vi "BPSK QPSK Simulation.vi"() -> ()   [LabVIEW 2013]
uses:
  <vilib>/addons/Modulation/Digital/General/MT Generate Bits (Galois, PN Order).vi
  <vilib>/addons/Modulation/Digital/General/MT Generate PSK System Parameters(M).vi
  <vilib>/addons/Modulation/Digital/General/MT Generate PSK Synchronization Parameters (bit array).vi
  <vilib>/addons/Modulation/Digital/General/MT Format Eye Diagram (complex).vi
  <vilib>/addons/Modulation/niDMT.lvlib
panel:
  out "recovered bits":i32[](array[numeric])
  out "transmitted bits":i32[](array[numeric])
  in  "stop":bool
  out "eye diagram":cluster{"t0":dbl, "dt":dbl, "Y":dbl[]}[](graph)
  out "baseband waveform":cluster{"t0":dbl, "dt":dbl, "Y":dbl[]}(graph)
  out "LED Array":cluster{bool[], bool[]}
  out "constellation graph":T1(graph)
  out "measurements":T2 {"phase offset (deg)" format="%.2f"; "frequency drift (Hz)" format="%.2f"; "frequency offset (Hz)" format="%.2f"}
  out "sync found index (symbols)":dbl format="%.4f"
  in  "Eb/N0 (10 dB)":dbl(slide)=10.0 scale=0.0..500.0
  in  "modulation type":T3(ring)
  in  "pulse shaping filter (none)":T4(ring)
  in  "M-FSK (4)":i32=2 caption="M-FSK (2)"
  in  "Message Bits":i32=128 caption="Message bits"
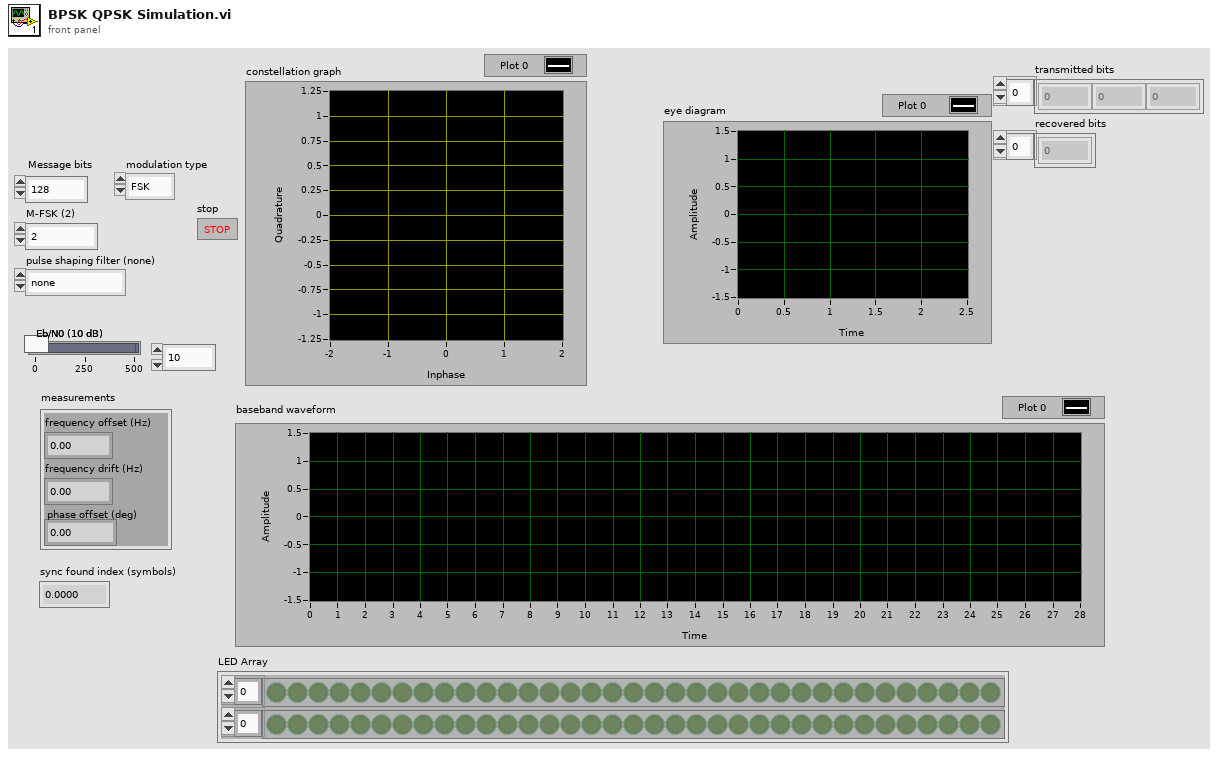
[diagram p1: front panel]
types:
  T1 = cluster{"constellation":dbl[], "oversampled data":dbl[]}[]
  T2 = cluster{"frequency offset (Hz)":dbl, "frequency drift (Hz)":dbl, "phase offset (deg)":dbl}
  T3 = enum16{"FSK", "PSK", "QAM", "MSK", "PAM", "ASK", "CPM"}
  T4 = enum16{"none", "Raised Cosine", "Root Raised Cos", "Gaussian"}
  T5 = cluster{"samples per symbol (16)":i32, "symbol map":cdb[], "differential PSK":enum16{"disable", "enable"}, "PSK type":u16}
  T6 = typedef "niAMT.lvlib/Complex Data Waveform.ctl" = cluster{"t0":dbl, "dt":dbl, "Y":cdb[]}
  T7 = cluster{"expected sync location (symbols)":i32, "sync sequence":cdb[], "sync location uncertainty (symbols)":i32, "sync indent (symbols)":i32}
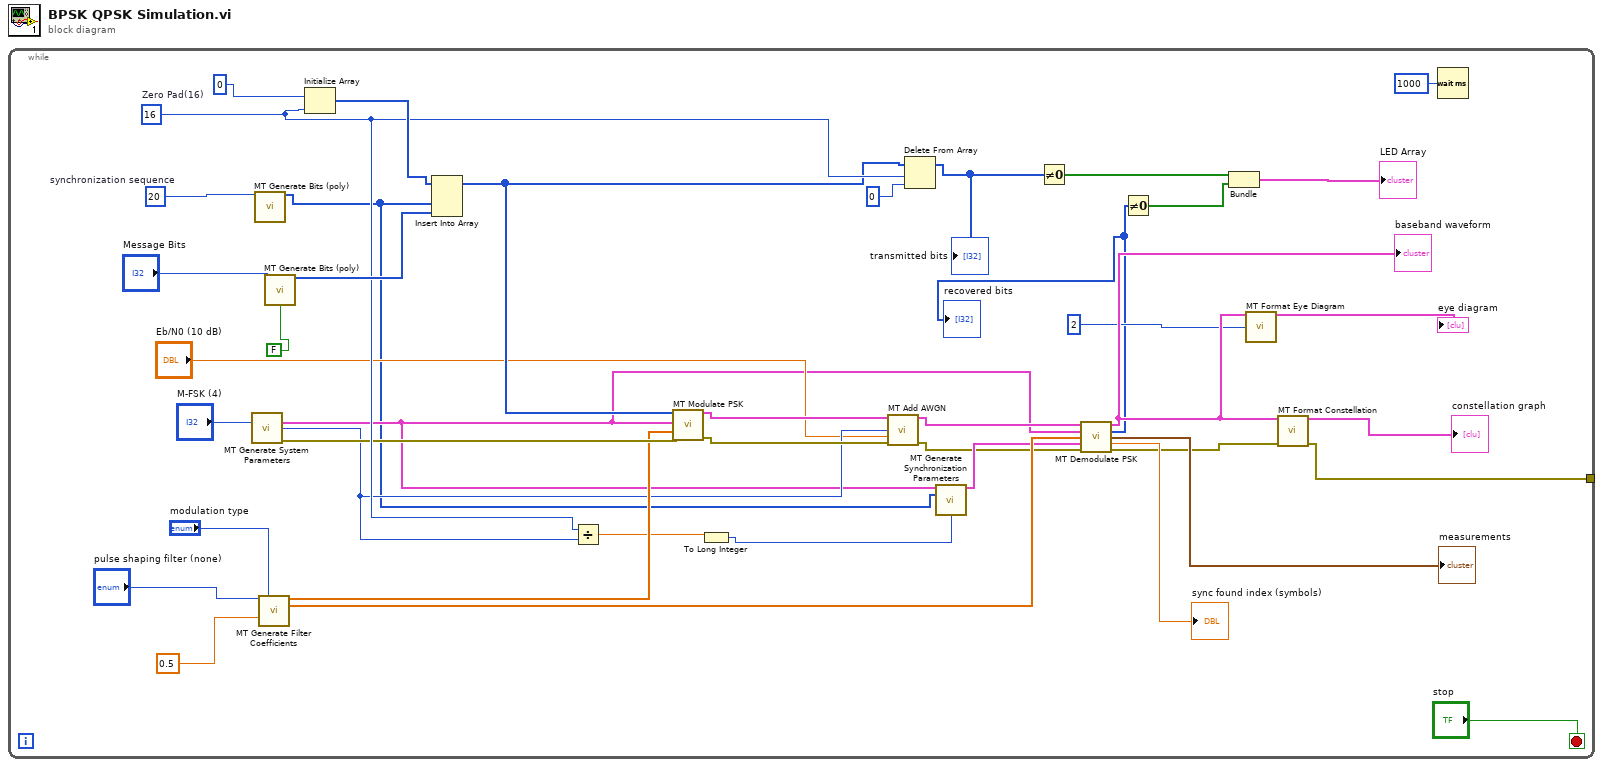
[diagram p0: block diagram]
diagram:
  n1 = while {
    tunnel: [w3] -> _
    stop <- "stop" stop-if-true
    w40 = 20  # synchronization sequence
    w28 = 16  # Zero Pad(16)
    n2 = call-poly <vilib>:"MT Generate System Parameters.vi"("M-PSK (4)"="M-FSK (4)") -> ("PSK system parameters"=w16:T5, "bits per symbol"=w22:i32, "error out"=w27:errorcluster)  [unwired: 12 in]
    n3 = call-poly <vilib>:"MT Generate Bits (poly).vi"("total bits (128)"=w40) -> ("output bit stream"=w15:i8[])  [unwired: 12 in, 2 out]
    n4 = call <vilib>:"MT Generate Filter Coefficients.vi"("pulse shaping filter (none)"="pulse shaping filter (none)", "modulation type"="modulation type", "filter parameter"=0.5) -> ("pulse shaping filter coefficients"=w26:dbl[], "matched filter coefficients"=w19:dbl[])  [unwired: 10 in, 1 out]
    n5 = call-poly <vilib>:"MT Generate Bits (poly).vi"("total bits (128)"="Message Bits", "reset? (T)"=FALSE) -> ("output bit stream"=w37:i8[])  [unwired: 11 in, 2 out]
    n6 = Initialize Array "Initialize Array"(0, w28) -> (w41:i32[])
    n7 = Insert Into Array "Insert Into Array"(array=w41, new element #1=w15, new element #2=w37) -> (w24:i32[])  [unwired: 1 in]
    n8 = Divide(x=w28, y=w22) -> (x/y=w18:dbl)
    n9 = call <vilib>:"MT Modulate PSK.vi"("input bit stream"=w24, "PSK system parameters"=w16, "pulse shaping filter coefficients"=w26, "error in (no error)"=w27) -> ("output complex waveform"=w25:T6, "error out"=w23:errorcluster)  [unwired: 9 in, 1 out]
    n10 = To Long Integer(number=w18) -> (32bit integer=w17:i32)
    n11 = call <vilib>:"MT Add AWGN.vi"("input complex waveform"=w25, "bits per symbol (1)"=w22, "Eb/N0 (10 dB)"="Eb/N0 (10 dB)", "error in (no error)"=w23) -> ("output complex waveform"=w20:T6, "error out"=w13:errorcluster)  [unwired: 9 in, 1 out]
    n12 = Delete From Array "Delete From Array"(array=w24, length=w28, index=0) -> (array with subset deleted=w35:i32[])  [unwired: 1 out]
    "transmitted bits" <- w35
    n13 = call-poly <vilib>:"MT Generate Synchronization Parameters.vi"("PSK system parameters"=w16, "sync bits"=w15, "sync location uncertainty (symbols)"=w17) -> ("PSK synchronization parameters"=w14:T7)  [unwired: 11 in, 1 out]
    n14 = Not Equal To 0?(x=w35) -> (x != 0?=w34:bool[])
    n15 = call <vilib>:"MT Demodulate PSK.vi"("input complex waveform"=w20, "PSK system parameters"=w16, "matched filter coefficients"=w19, "synchronization parameters"=w14, "error in (no error)"=w13) -> ("recovered complex waveform"=w6:T6, "output bit stream"=w1:i8[], "measurements"=→"measurements":T2, "sync found index (symbols)"=→"sync found index (symbols)":dbl, "error out"=w10:errorcluster)  [unwired: 6 in]
    "baseband waveform" <- w6
    "recovered bits" <- w1
    n16 = Not Equal To 0?(x=w1) -> (x != 0?=w8:bool[])
    n17 = Bundle "Bundle"(w34, w8) -> (→"LED Array":cluster{bool[], bool[]})  [unwired: 1 in]
    n18 = call-poly <vilib>:"MT Format Eye Diagram.vi"("waveform"=w6, "eye length"=2) -> ("eye diagram"=→"eye diagram":cluster{"t0":dbl, "dt":dbl, "Y":dbl[]}[])  [unwired: 12 in, 1 out]
    n19 = call <vilib>:"MT Format Constellation.vi"("waveform"=w6, "error in (no error)"=w10) -> ("constellation graph"=→"constellation graph":T1, "error out"=w3:errorcluster)  [unwired: 12 in]
    n20 = Wait (ms)(milliseconds to wait=u32 1000) -> ()  [unwired: 1 out]
  }
